vi "Read Msg Output.vi"(10 "Msg Output":refnum<class "Msg Output.lvclass">) -> ()   [LabVIEW 2025, in "jettl.lvlib" / "Stopped Msg.lvlib" / "Stopped Msg Output.lvclass"]
uses:
  Stopped Msg Output.lvclass
  Msg Output/Msg Output.lvclass
  Stopped Msg Output.lvclass/Stopped Msg Output.ctl
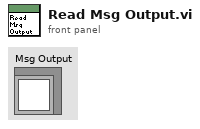
[diagram p1: front panel]
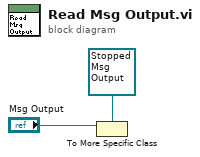
[diagram p0: block diagram]
diagram:
  n1 = To More Specific Class(target class=refnum<class "Stopped Msg Output.lvclass"> refnum ("jettl.lvlib:Stopped Msg.lvlib:Stopped Msg Output.lvclass"), reference="Msg Output") -> ()  [unwired: 1 in, 2 out]
